vi "Parse Country Code.vi"(4 "Country":T1=enum."Germany") -> (1 "Country Code":string)   [LabVIEW 2025, in "Geocoding Actor.lvlib" / "Geocoding.lvclass"]
uses:
  Geocoding.lvclass
  Country.ctl
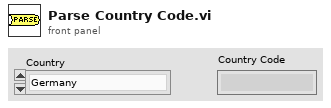
[diagram p1: front panel]
types:
  T1 = typedef "Geocoding Actor.lvlib/Geocoding.lvclass/Country.ctl" = enum16{"Austria", "Germany", "Switzerland"}
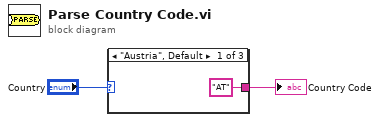
[diagram p0: block diagram]
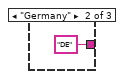
[diagram p2: hidden frame]
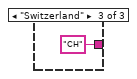
[diagram p3: hidden frame]
diagram:
  n1 = case shown="\"Austria\", Default" "Country" {
    tunnel: ["AT" ("Country Code") "DE" ("Country Code") "CH" ("Country Code")] -> w1
    frame "Austria", Default {
    }
    frame "Germany" {
    }
    frame "Switzerland" {
    }
  }
  "Country Code" <- w1
